vi "ReadSpectrum(SubVI)-ALL.vi"(10 "Continuous \nStrobe Delay":i32, 11 "Enter the \nInetegration Time":i32) -> (1 "Spectrum Values":dbl[](array[numeric]), 2 "WL Values":dbl[](array[numeric]), 3 "Number of Spectrometers":i32)   [LabVIEW 2020]
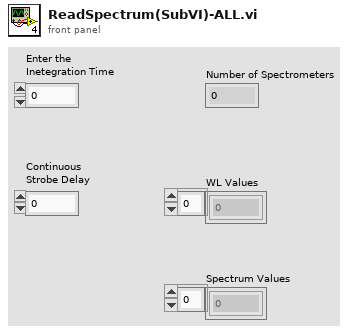
[diagram p1: front panel]
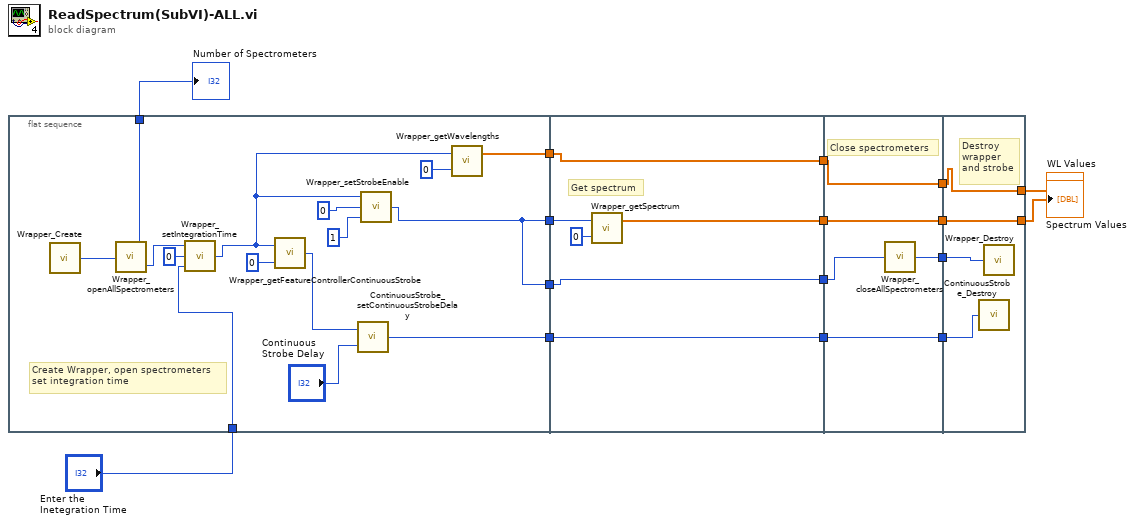
[diagram p0: block diagram]
diagram:
  n1 = flat-sequence {
    tunnel: [w21] -> w16
    tunnel: [w20] -> w15
    tunnel: [w20] -> w14
    tunnel: [w19] -> w13
    tunnel: "Enter the \nInetegration Time" -> [w18]
    tunnel: [w17] -> w4
    tunnel: [w37] -> w12
    tunnel: w16 -> [w37]
    tunnel: w15 -> [w36]
    tunnel: w14 -> [w34]
    tunnel: [w34] -> w11
    tunnel: w13 -> [w33]
    tunnel: [w33] -> w10
    tunnel: [w32] -> w9
    tunnel: [w42] -> w8
    tunnel: w12 -> [w42]
    tunnel: w11 -> [w41]
    tunnel: [w40] -> w7
    tunnel: [w39] -> w6
    tunnel: w10 -> [w39]
    tunnel: [w38] -> w5
    tunnel: w9 -> [w38]
    tunnel: w8 -> [w46]
    tunnel: w7 -> [w45]
    tunnel: [w44] -> w1
    tunnel: w6 -> [w44]
    tunnel: [w43] -> w2
    tunnel: w5 -> [w43]
    frame #0 {
      # "Create Wrapper, open spectrometers\nset integration time"
      n2 = call "Wrapper_Create.vi"() -> ("Wrapper"=w31:u32)
      n3 = call "Wrapper_openAllSpectrometers.vi"("Wrapper In"=w31) -> ("Number of Spectrometers"=w17:i32, "Wrapper Out"=w24:u32)
      n4 = call "Wrapper_setIntegrationTime.vi"("Integration Time"=w18, "Spectrometer Index"=0 ("Index"), "Wrapper In"=w24) -> ("Wrapper Out"=w22:u32)
      n5 = call "Wrapper_getFeatureControllerContinuousStrobe.vi"("Index"=0, "Wrapper"=w22) -> ("ContinuousStrobe"=w28:u32)
      n6 = call "ContinuousStrobe_setContinuousStrobeDelay.vi"("delay"="Continuous \nStrobe Delay", "ContinuousStrobe In"=w28) -> ("ContinuousStrobe Out"=w21:u32)
      n7 = call "Wrapper_setStrobeEnable.vi"("On/Off"=1, "Index"=0, "Wrapper In"=w22) -> ("Wrapper Out"=w20:u32)
      n8 = call "Wrapper_getWavelengths.vi"("Index"=0, "Wrapper"=w22) -> ("WL Values"=w19:dbl[])  [unwired: 1 out]
    }
    frame #1 {
      # "Get spectrum"
      n9 = call "Wrapper_getSpectrum.vi"("Index"=0, "Wrapper"=w36) -> ("Spectrum Values"=w32:dbl[])  [unwired: 1 out]
    }
    frame #2 {
      # "Close spectrometers"
      n10 = call "Wrapper_closeAllSpectrometers.vi"("Wrapper In"=w41) -> ("Wrapper Out"=w40:u32)
    }
    frame #3 {
      # "Destroy \nwrapper \nand strobe"
      n11 = call "ContinuousStrobe_Destroy.vi"("ContinuousStrobe"=w46) -> ()
      n12 = call "Wrapper_Destroy.vi"("Wrapper"=w45) -> ()
    }
  }
  "Number of Spectrometers" <- w4
  "Spectrum Values" <- w2
  "WL Values" <- w1
